vi "CalcBatteryRunTime.vi"(8 "Error In":errorcluster, 9 "Mode":T1(ring), 10 "Enviroment Info":variant, 11 "BattleDroid In":refnum<class "BattleDroid.lvclass">) -> (0 "Error Out":errorcluster, 2 "Battery RunTime":u64, 3 "BattleDroid Out":refnum<class "BattleDroid.lvclass">)   [LabVIEW 2021, in "BattleDroid.lvclass"]
uses:
  BattleDroid.lvclass
  <vilib>/numeric/Random Number (Range) U64.vi
  <vilib>/numeric/sub_Random U32.vi
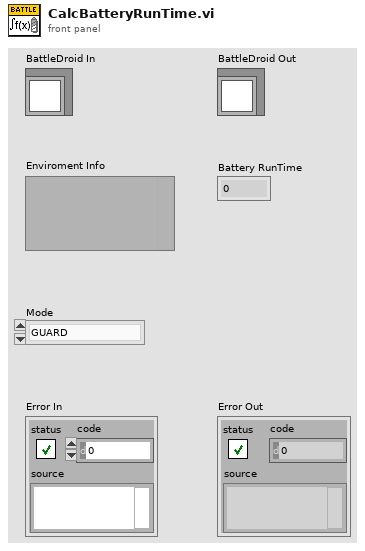
[diagram p1: front panel]
types:
  T1 = enum16{"GUARD", "RECON", "ATTACK ", "MAINTAINCE"}
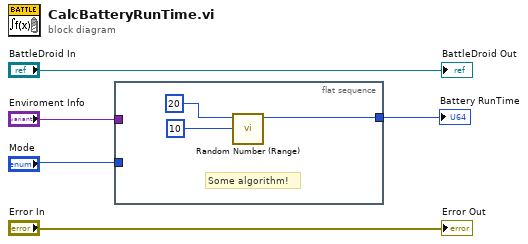
[diagram p0: block diagram]
diagram:
  n1 = flat-sequence {
    tunnel: "Enviroment Info" -> [_]
    tunnel: "Mode" -> [_]
    tunnel: [w6] -> w1
    frame #0 {
      # "Some algorithm!"
      n2 = call-poly <vilib>:"Random Number (Range).vi"("lower bound (0)"=u64 10, "upper bound (100)"=u64 20) -> ("number"=w6:u64)  [unwired: 9 in]
    }
  }
  "Error Out" <- "Error In"
  "BattleDroid Out" <- "BattleDroid In"
  "Battery RunTime" <- w1
